vi "Mock Stop Helper Loop.vi"(8 "error in (no error)":errorcluster, 11 "Mock Process in":refnum<class "Mock Process.lvclass">) -> (0 "error out":errorcluster, 3 "Mock Process out":refnum<class "Mock Process.lvclass">)   [LabVIEW 2020, in "Mock Process.lvclass"]
uses:
  Mock Process.lvclass
  C:/git/astemes-triarc-framework/source/Framework/Helper Loop/Helper Loop.lvclass
  Framework/Process/Process.lvclass/Process.ctl
  Framework/Process/Public/Lifecycle/Get Lifecycle State.vi
  <vilib>/Utility/error.llb/Clear Errors.vi
  <vilib>/Utility/error.llb/Error Cluster From Error Code.vi
  Framework/Process/Process.lvclass
  Framework/Helper Loop/Helper Loop.lvclass
  Mock Process.lvclass/Mock Process.ctl
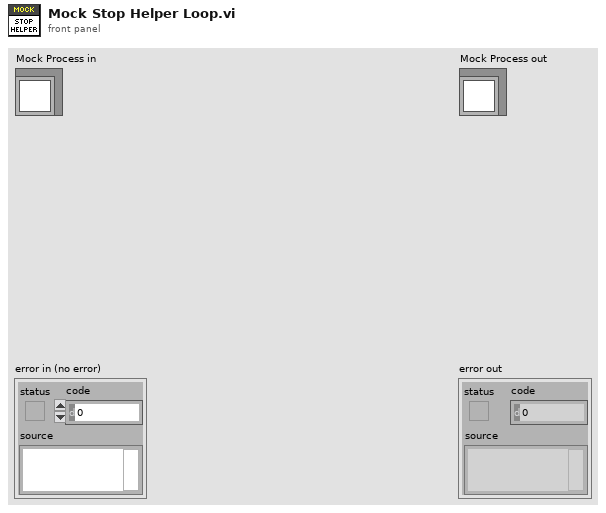
[diagram p1: front panel]
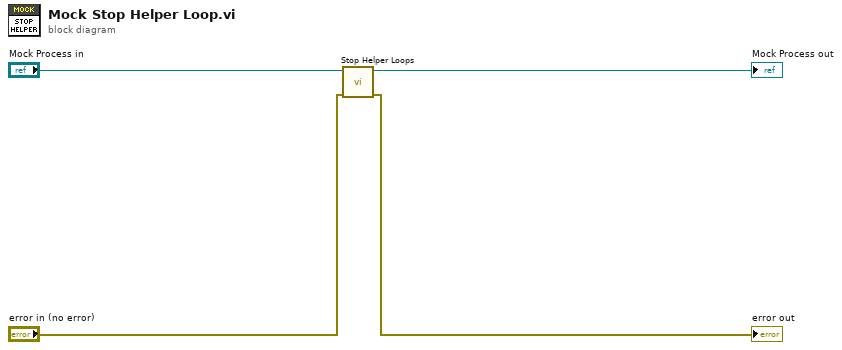
[diagram p0: block diagram]
diagram:
  n1 = call "Stop Helper Loops.vi"("error in (no error)"="error in (no error)", "Helper Loop In"="Mock Process in") -> ("error out"=→"error out":errorcluster, "Helper Loop Out"=→"Mock Process out":refnum<class "Mock Process.lvclass">)  [unwired: 8 in]
